vi "Mimic 3.vi"() -> ()   [LabVIEW 2018]
uses:
  <vilib>/Utility/file.llb/Write Delimited Spreadsheet (DBL).vi
panel:
  out "BRNR FLNG TMP":dbl format="%.1f"
  out "DIL FLG TMP 4":dbl format="%.1f"
  out "DIL FLG TMP 3":dbl format="%.1f"
  out "DIL FLG TMP 2":dbl format="%.1f"
  out "EX GAS TMP":dbl format="%.1f"
  out "DIL FLG TMP":dbl format="%.1f"
  out "ADPT FLG TMP":dbl format="%.1f"
  out "WTR INLT TMP":dbl format="%.1f"
  out "BRNR FC 4":dbl format="%.1f"
  out "BRNR FC 3":dbl format="%.1f"
  out "BRNR FC 2":dbl format="%.1f"
  out "EQ Ratio":dbl format="%_3f"
  out "PRI AFR":dbl format="%_3f"
  out "BRNR dp":dbl format="%.1f"
  out "Primary TMP":dbl format="%.1f"
  out "Combustion Pres.":dbl format="%.1f"
  out "Plume Pres.":dbl format="%.1f"
  out "Bypass Flow":dbl format="%.1f"
  out "TBC TMP":dbl format="%.1f"
  in  "Chamber 4 Threshold":dbl
  in  "Chamber 3 Threshold":dbl
  in  "Chamber 2 Threshold":dbl
  in  "Chamber 1 Threshold":dbl
  out "WTR BPVP":dbl format="%.1f"
  out "WTR BPVB":dbl format="%.1f"
  out "WTR BPVT":dbl format="%.1f"
  out "WTR P":dbl format="%.1f"
  out "WTR TMP 2":dbl format="%.1f"
  out "WTR TMP 1":dbl format="%.1f"
  out "WTR PL1":dbl format="%.1f"
  out "WTR GAUP":dbl format="%.1f"
  out "WTR GADW":dbl format="%.1f"
  out "WIN TMP":dbl format="%.1f"
  out "Flame status light":bool
  in  "Flame On":bool
  in  "Record Button":bool
  in  "Filename":path=path "C:/Users/dotta/OneDrive/Desktop/Labview Projs/Mimic/test write 1.xlsx"
  in  "?":bool
  in  "Refresh Rate (ms)":u32
  out "Current Date/time":timestamp format="%<%I:%M:%S %p\n%d/%m/%y>T"
  out "Pres 5 [bar]":dbl format="%.1f"
  out "Temp 5 [c]":dbl format="%.1f"
  out "Flow 5 [g/s]":dbl format="%.1f"
  out "Pres 4 [bar]":dbl format="%.1f"
  out "Temp 4 [c]":dbl format="%.1f"
  out "Flow 4 [g/s]":dbl format="%.1f"
  out "Pres 3 [bar]":dbl format="%.1f"
  out "Temp 3 [c]":dbl format="%.1f"
  out "Flow 3 [g/s]":dbl format="%.1f"
  out "Pres 2 [bar]":dbl format="%.1f"
  out "Temp 2 [c]":dbl format="%.1f"
  out "Flow 2 [g/s]":dbl format="%.1f"
  out "Pres 1 [bar]":dbl format="%.1f"
  out "Temp 1 [c]":dbl format="%.1f"
  out "Flow 1 [g/s]":dbl format="%.1f"
  out "CMB EX TMP":dbl format="%.1f"
  out "GA GAS TM":dbl format="%.1f"
  out "TUBE 1":dbl format="%.1f"
  out "TUBE 2":dbl format="%.1f"
  out "LANCE TIP":dbl format="%.1f"
  out "BRNR NOZ":dbl format="%.1f"
  out "BRNR FC":dbl format="%.1f"
  # "HPOC HPGSB RIB COND"
  # "INLET"
  # "FLOW"
  # "[BAR]"
  # "[mB]"
  # "BAR"
  # "[c]"
  # "RIG"
  # "[c]"
  # "[c]"
  # "[c]"
  # "[c]"
  # "[c]"
  # "[g/s]"
  # "[c]"
  # "[c]"
  # "[g/s]"
  # "[c]"
  # "[c]"
  # "[c]"
  # "[g/s]"
  # "[c]"
  # "[c]"
  # "[c]"
  # "[c]"
  # "[c]"
  # "[c]"
  # "[c]"
  # "[c]"
  # "[c]"
  # "[c]"
  # "[c]"
  # "Line 5"
  # "Line 4"
  # "Line 3"
  # "Line 2"
  # "Line 1"
  # "[c]"
  # "[c]"
  # "[c]"
  # "[c]"
  # "[c]"
  # "[c]"
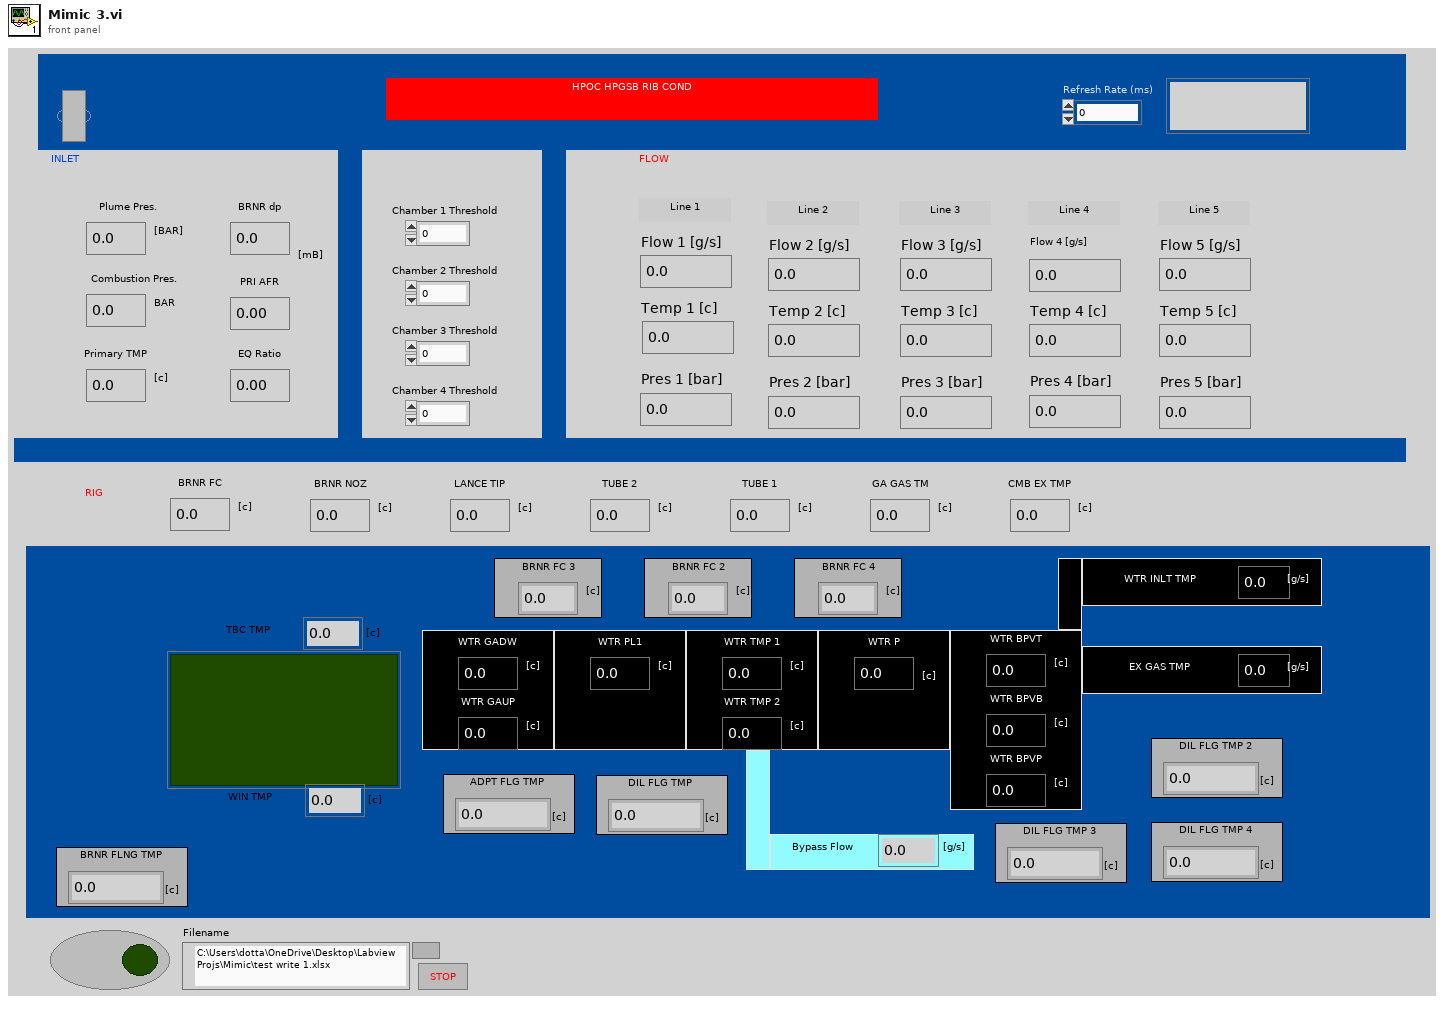
[diagram p1: front panel]
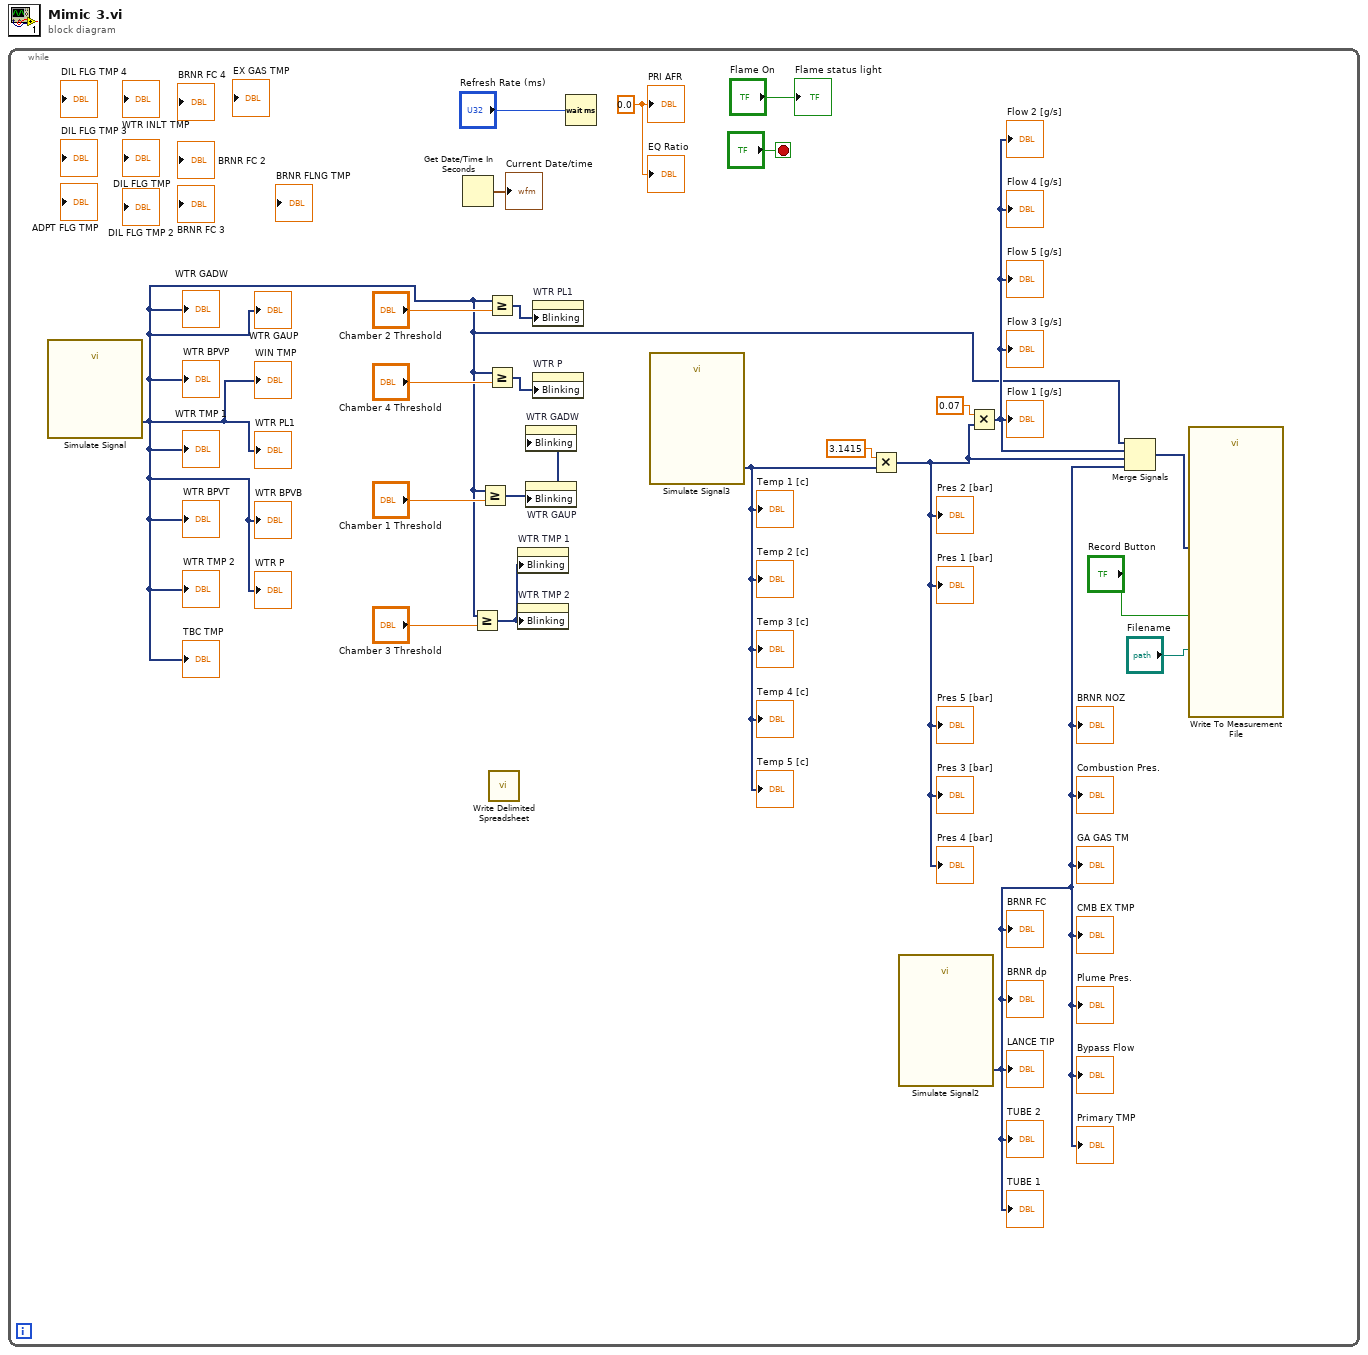
[diagram p0: block diagram]
diagram:
  n1 = while {
    stop <- "?" stop-if-true
    w5 = 0.0 ("PRI AFR")
    n2 = call "Simulate Signal"() -> ("Sine"=w1:dynamicdata)  [unwired: 14 in, 1 out]
    "WIN TMP" <- w1
    "WTR GADW" <- w1
    "WTR GAUP" <- w1
    "WTR PL1" <- w1
    "WTR TMP 1" <- w1
    "WTR TMP 2" <- w1
    "WTR P" <- w1
    "WTR BPVT" <- w1
    "WTR BPVB" <- w1
    "WTR BPVP" <- w1
    "TBC TMP" <- w1
    n3 = Get Date/Time In Seconds() -> (seconds since 1Jan1904=→"Current Date/time":timestamp)
    n4 = Greater Or Equal?(x=w1, y="Chamber 3 Threshold") -> (x >= y?=w8:dynamicdata)
    n5 = Greater Or Equal?(x=w1, y="Chamber 1 Threshold") -> (x >= y?=w12:dynamicdata)
    n6 = Greater Or Equal?(x=w1, y="Chamber 2 Threshold") -> (x >= y?=w11:dynamicdata)
    n7 = Greater Or Equal?(x=w1, y="Chamber 4 Threshold") -> (x >= y?=w6:dynamicdata)
    n8 = call-poly <vilib>:"Write Delimited Spreadsheet.vi"() -> ()  [unwired: 14 in, 2 out]
    n9 = property on="WTR TMP 1" class="DigNum (strict)"("Blinking"=w8) -> ()  [unwired: 2 in, 2 out]
    n10 = property on="WTR TMP 2" class="DigNum (strict)"("Blinking"=w8) -> ()  [unwired: 2 in, 2 out]
    n11 = property on="WTR GADW" class="DigNum (strict)"("Blinking"=w12) -> ()  [unwired: 2 in, 2 out]
    n12 = property on="WTR GAUP" class="DigNum (strict)"("Blinking"=w12) -> ()  [unwired: 2 in, 2 out]
    n13 = property on="WTR PL1" class="DigNum (strict)"("Blinking"=w11) -> ()  [unwired: 2 in, 2 out]
    n14 = property on="WTR P" class="DigNum (strict)"("Blinking"=w6) -> ()  [unwired: 2 in, 2 out]
    n15 = Wait (ms)(milliseconds to wait="Refresh Rate (ms)") -> ()  [unwired: 1 out]
    n16 = call "Simulate Signal3"() -> ("Sine with Uniform Noise"=w21:dynamicdata)  [unwired: 14 in, 1 out]
    "Temp 1 [c]" <- w21
    "Temp 2 [c]" <- w21
    "Temp 3 [c]" <- w21
    "Temp 4 [c]" <- w21
    "Temp 5 [c]" <- w21
    n17 = Multiply(x=3.1415 ("x*y"), y=w21) -> (x*y=w3:dynamicdata)
    "Pres 1 [bar]" <- w3
    "Pres 2 [bar]" <- w3
    "Pres 3 [bar]" <- w3
    "Pres 4 [bar]" <- w3
    "Pres 5 [bar]" <- w3
    n18 = call "Simulate Signal2"() -> ("Sine with Uniform Noise"=w4:dynamicdata)  [unwired: 14 in, 1 out]
    "BRNR FC" <- w4
    "BRNR NOZ" <- w4
    "LANCE TIP" <- w4
    "TUBE 2" <- w4
    "TUBE 1" <- w4
    "GA GAS TM" <- w4
    "CMB EX TMP" <- w4
    "Plume Pres." <- w4
    "Combustion Pres." <- w4
    "Primary TMP" <- w4
    "BRNR dp" <- w4
    "Bypass Flow" <- w4
    n19 = Multiply(x=0.07 ("x*y"), y=w3) -> (x*y=w2:dynamicdata)
    "Flow 1 [g/s]" <- w2
    "Flow 2 [g/s]" <- w2
    "Flow 3 [g/s]" <- w2
    "Flow 4 [g/s]" <- w2
    "Flow 5 [g/s]" <- w2
    n20 = Merge Signals(w1, w2, w3, w4) -> (w15:dynamicdata)
    n21 = call "Write To Measurement File"("Signals"=w15, "Enable"="Record Button", "Filename"="Filename") -> ()  [unwired: 14 in, 3 out]
    "Flame status light" <- "Flame On"
    "PRI AFR" <- w5
    "EQ Ratio" <- w5
  }
